vi "Pressure_3_R1.vi"() -> ()   [LabVIEW 2020]
uses:
  Support/Controls/Cmd_Mouse Popup.ctl
  Support/Controls/Clst_Initialize Input.ctl
  Support/Controls/Clst_Result inspec.ctl
  Support/Controls/Cmd_Var Data IO.ctl
  Variables/Global_Cal Info.vi
panel:
  in  "기준온도":string="15" caption="유체기준온도"
  in  "유체":string(combo)="담수"
  in  "Measured_ADJ":string[][](table) caption="Measured (조정후)"
  out "최고수심 (m)":string
  out "Form":string[][](table)
  in  "교정방법":string(combo)="기본교정"
  out "Resolution":string[][](table) caption="Spec"
  in  "지시형태":string(combo)="Check"
  in  "Spec 변경":bool
  in  "Random":bool
  out "Spec":string[][](table)
  out "제목":string
  out "에러 출력":errorcluster
  out "Condition":string[][](table)
  in  "최소눈금 (m)":string(combo)
  out "최대용량 (kPa)":string
  in  "Measured":string[][](table) caption="Measured (조정전)"
  out "Load?":bool
  # "℃"
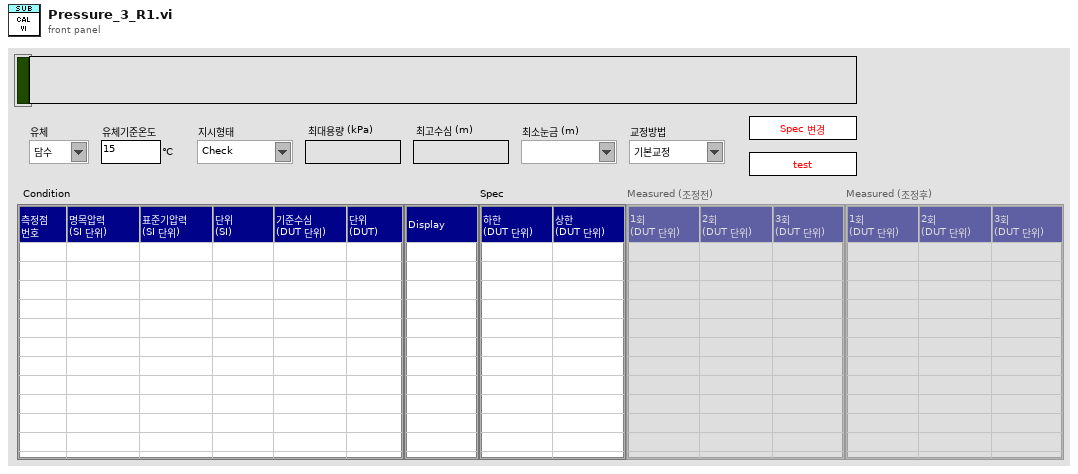
[diagram p1: front panel]
types:
  T1 = typedef "Cmd_Mouse Popup.ctl" = enum16{"활성화", "메뉴선택"}
  T2 = cluster{"Shift":bool, "Ctrl":bool, "Alt":bool, "Cmd":bool, "Opt":bool}
  T3 = enum8{"Enabled", "Disabled", "Disabled and Grayed Out"}
  T4 = cluster{"DisabledEnum":enum8{"Enabled", "Disabled", "Disabled and Grayed Out"}, "Value":string[][], "DisabledEnum":enum8{"Enabled", "Disabled", "Disabled and Grayed Out"}, "Value":string[][], "지시형태":string}
  T5 = typedef "Clst_Initialize Input.ctl" = cluster{"Initialize 1":cluster{"Condition":refnum<vi>[], "Spec":refnum<vi>[], "Measured":refnum<vi>[], "Resolution":refnum<vi>[], "Func_ext":string, "제목":refnum<vi>, "Measured_ADJ":refnum<vi>[]}, "Initialize 2":cluster{"문자열":refnum<vi>[], "콤보박스":refnum<vi>[], "링":refnum<vi>[], "열거형":refnum<vi>[], "테이블":refnum<vi>[], "여러열":refnum<vi>[], "디지털(DBL)":refnum<vi>[], "3D string":refnum<vi>[], "ctrl":refnum<vi>[], "boolean":refnum<vi>[]}}
  T6 = typedef "Clst_Result inspec.ctl" = cluster{"분해능":string, "문자열 1":string, "문자열 2":string, "숫자형 1":i32, "숫자형 2":i32, "숫자형 3":dbl, "문자배열 1D":string[], "문자배열 2D":string[][], "문자배열 3D":string[][][], "문자배열 4D":string[][][][], "불리언 1D":bool[]}
  T7 = typedef "Cmd_Var Data IO.ctl" = enum16{"Condition", "Condition Default", "Condition_Temp", "Resolution", "Resolution Default", "Resolution Old", "Spec", "Spec Default", "Spec Old", "Spec Temp", "Result", "Result2", "Result3", "Result_Temp", "Result_ADJ", "Result_ADJ2", "STD1", "STD2", "STD3", "STD4", "STD5", "STD Temp", "CMC", "CMC Default"}
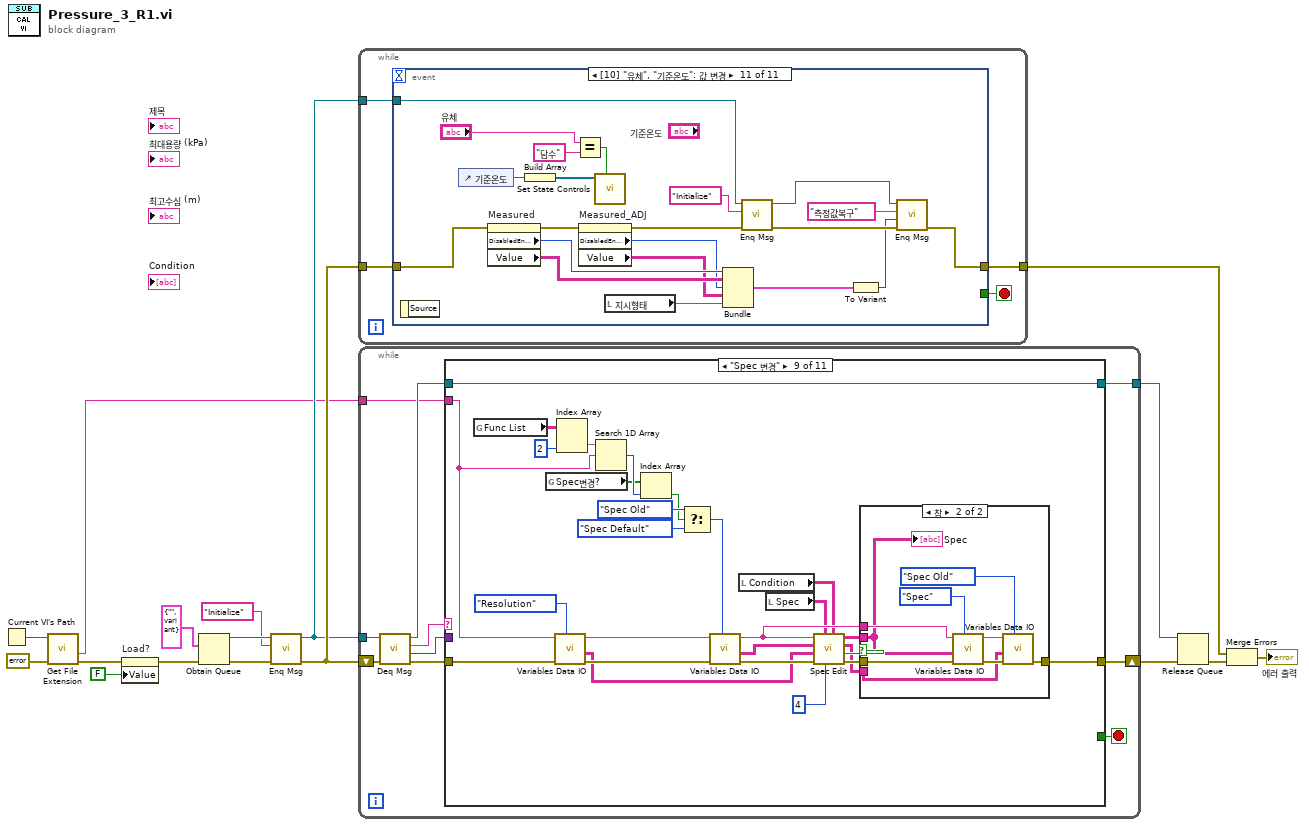
[diagram p0: block diagram]
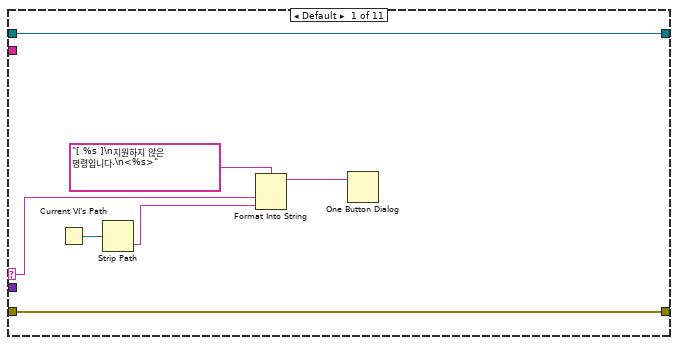
[diagram p2: hidden frame]
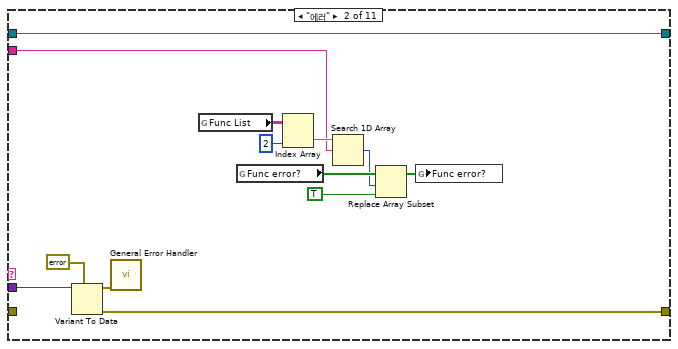
[diagram p3: hidden frame]
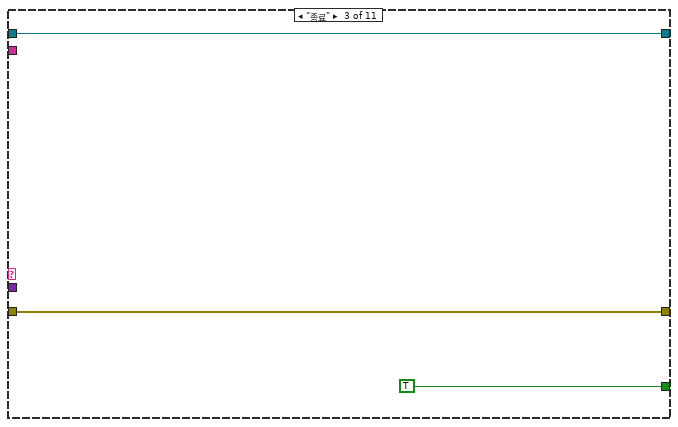
[diagram p4: hidden frame]
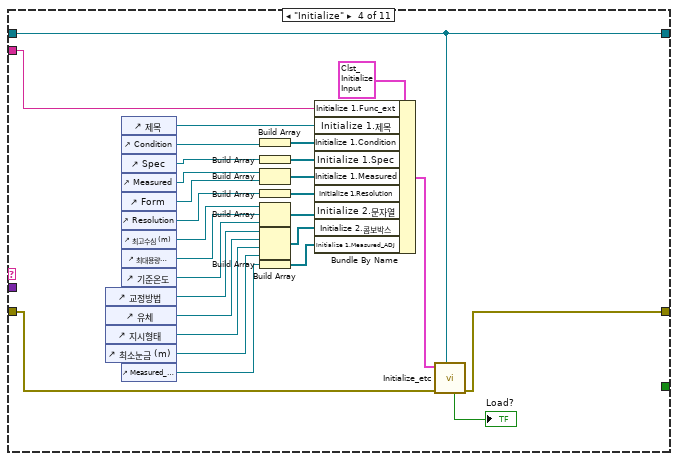
[diagram p5: hidden frame]
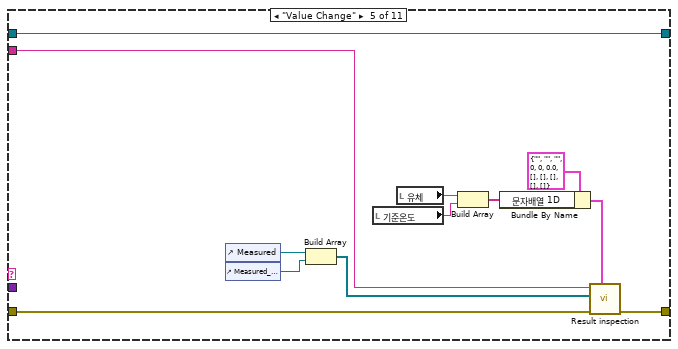
[diagram p6: hidden frame]
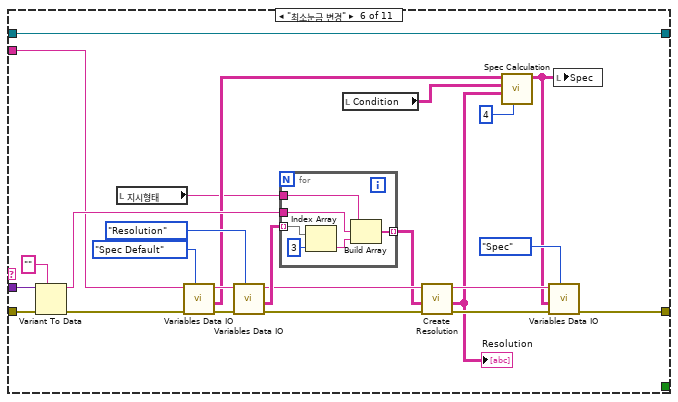
[diagram p7: hidden frame]
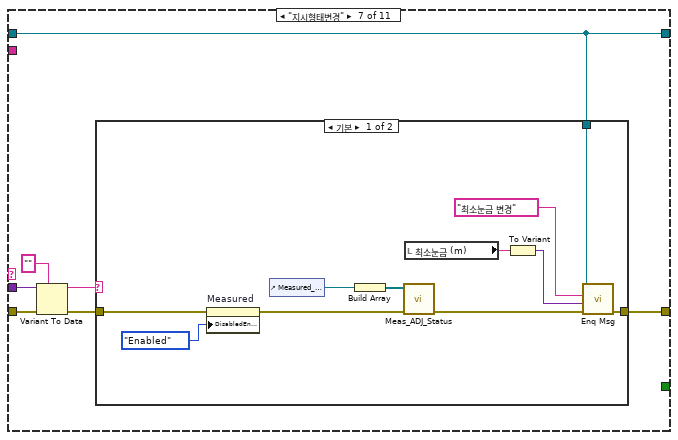
[diagram p8: hidden frame]
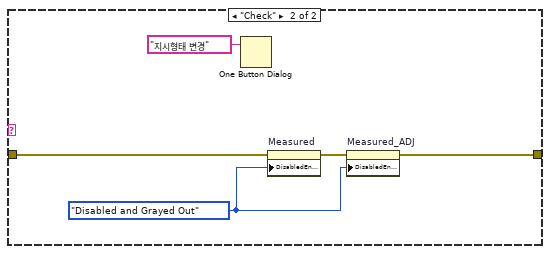
[diagram p9: hidden frame]
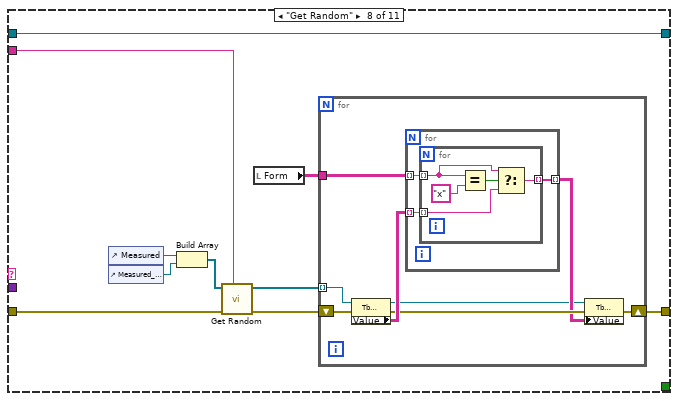
[diagram p10: hidden frame]
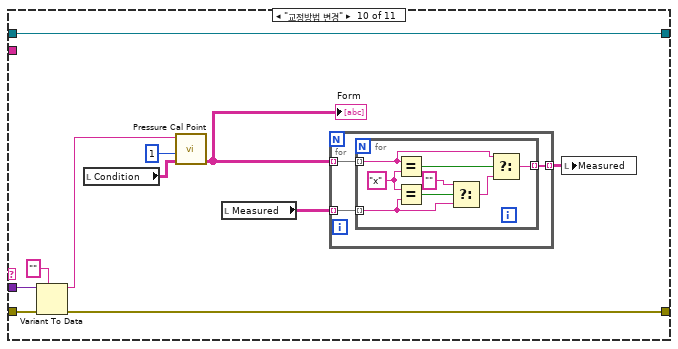
[diagram p12: hidden frame]
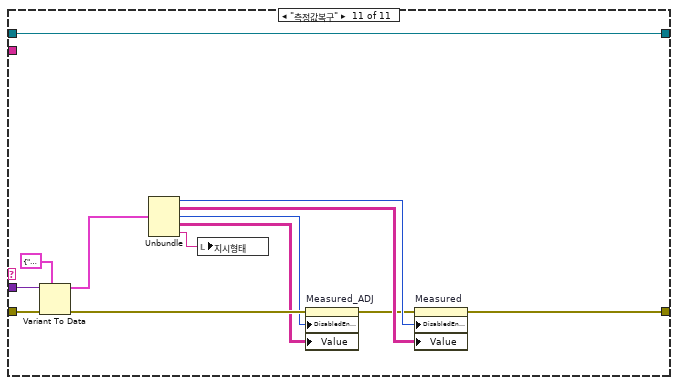
[diagram p13: hidden frame]
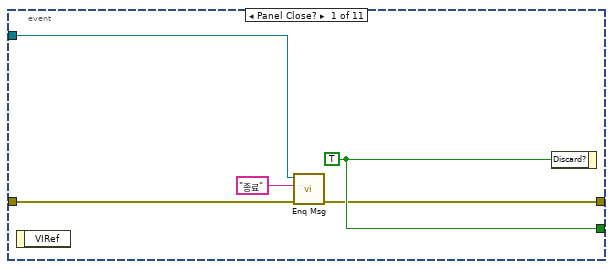
[diagram p14: hidden frame]
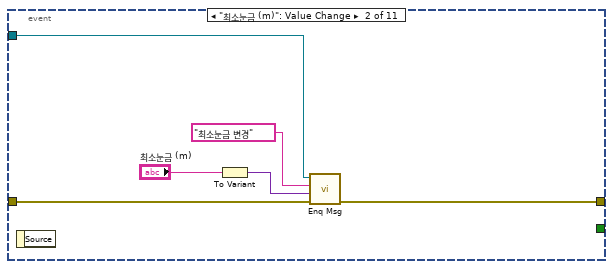
[diagram p15: hidden frame]
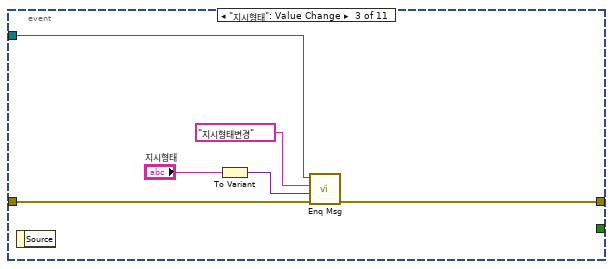
[diagram p16: hidden frame]
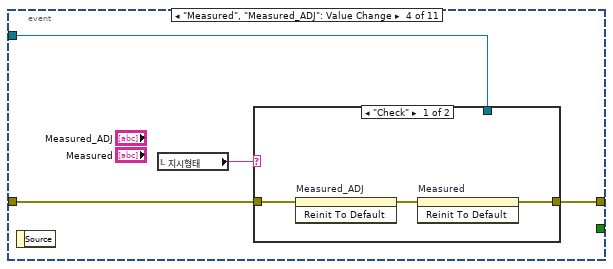
[diagram p17: hidden frame]
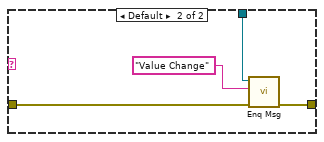
[diagram p18: hidden frame]
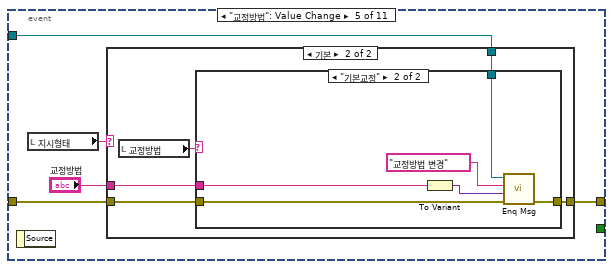
[diagram p19: hidden frame]
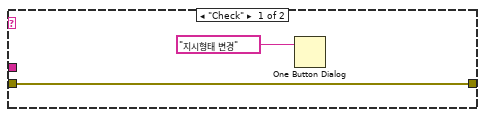
[diagram p20: hidden frame]
diagram:
  n1 = Current VI's Path() -> (path=w5:path)
  n2 = call <vilib>:"Get File Extension.vi"("error in (no error)"=errorcluster {"status"=FALSE, "code"=0, "source"=""} ("에러 상수"), "file"=w5) -> ("error out"=w2:errorcluster, "filename without extension"=w4:string)  [unwired: 5 in, 3 out]
  n3 = property on="Load?" class="Bool (엄격한)"(error in=w2, "Value"=FALSE ("Load?")) -> (error out=w1:errorcluster)  [unwired: 1 in, 1 out]
  n4 = Obtain Queue(element data type=cluster{"메세지":string, "값":variant} {"메세지"="", "값"=variant} ("Message Cluster"), error in (no error)=w1) -> (queue out=w14:refnum<queue>, error out=w16:errorcluster)  [unwired: 3 in, 1 out]
  n5 = call "Enq Msg.vi"("에러 입력(에러 없음)"=w16, "메세지"="Initialize", "큐 입력"=w14) -> ("에러 출력"=w15:errorcluster, "큐 출력"=w12:refnum<queue>)  [unwired: 7 in]
  n6 = while {
    tunnel: w15 -> [w19]
    tunnel: w12 -> [w20]
    tunnel: [w18] -> w9
    stop <- w21 stop-if-true
    n7 = event shown="[10] \"유체\", \"기준온도\": 값 변경" {
      selector: _ -> [_ _ _ _ _ _ _ _ _ _ _]
      dyn-events: _ -> [_ _ _ _ _ _ _ _ _ _ _]
      timeout: _ -> [_ _ _ _ _ _ _ _ _ _ _]
      tunnel: [w26 _ _ _ _ _ _ _ _ _ _] -> w21
      tunnel: w20 -> [w24 w31 w37 w41 w50 _ w90 _ w103 w109 w127]
      tunnel: w19 -> [w25 w32 w38 w42 w53 w86 w94 w101 w104 w111 w121]
      tunnel: [w22 w30 w36 w40 w54 w85 w89 w100 w102 w110 w124] -> w18
      event Panel Close? {
        w26 = TRUE ("버림?")
        n8 = event-data() -> ()  [unwired: 1 in, 1 out]
        n9 = call "Enq Msg.vi"("에러 입력(에러 없음)"=w25, "메세지"="종료", "큐 입력"=w24) -> ("에러 출력"=w22:errorcluster)  [unwired: 7 in, 1 out]
        n10 = event-data("Discard?"=w26) -> ()  [unwired: 1 in, 1 out]
      }
      event "최소눈금 (m)": Value Change {
        n11 = event-data() -> ()  [unwired: 1 in, 1 out]
        n12 = To Variant(anything="최소눈금 (m)") -> (Variant=w27:variant)
        n13 = call "Enq Msg.vi"("에러 입력(에러 없음)"=w32, "값"=w27, "메세지"="최소눈금 변경", "큐 입력"=w31) -> ("에러 출력"=w30:errorcluster)  [unwired: 6 in, 1 out]
      }
      event "지시형태": Value Change {
        n14 = event-data() -> ()  [unwired: 1 in, 1 out]
        n15 = To Variant(anything="지시형태") -> (Variant=w34:variant)
        n16 = call "Enq Msg.vi"("에러 입력(에러 없음)"=w38, "값"=w34, "메세지"="지시형태변경", "큐 입력"=w37) -> ("에러 출력"=w36:errorcluster)  [unwired: 6 in, 1 out]
      }
      event "Measured", "Measured_ADJ": Value Change {
        n17 = event-data() -> ()  [unwired: 1 in, 1 out]
        n18 = local read "지시형태"() -> (w39:string)
        n19 = case shown="\"Check\"" w39 {
          tunnel: w42 -> [w45 w49]
          tunnel: w41 -> [_ w48]
          tunnel: [w43 w47] -> w40
          frame "Check" {
            n20 = invoke on="Measured_ADJ" class="Tbl (엄격한)" method="Reinit To Default"(error in=w45) -> (error out=w44:errorcluster)  [unwired: 2 in, 2 out]
            n21 = invoke on="Measured" class="Tbl (엄격한)" method="Reinit To Default"(error in=w44) -> (error out=w43:errorcluster)  [unwired: 2 in, 2 out]
          }
          frame Default {
            n22 = call "Enq Msg.vi"("에러 입력(에러 없음)"=w49, "메세지"="Value Change", "큐 입력"=w48) -> ("에러 출력"=w47:errorcluster)  [unwired: 7 in, 1 out]
          }
        }
      }
      event "교정방법": Value Change {
        n23 = event-data() -> ()  [unwired: 1 in, 1 out]
        n24 = local read "지시형태"() -> (w51:string)
        n25 = case shown="기본" w51 {
          tunnel: w53 -> [w56 w61]
          tunnel: w50 -> [_ w60]
          tunnel: [w56 w59] -> w54
          tunnel: "교정방법" -> [_ w58]
          frame "Check" {
            n26 = One Button Dialog(message="지시형태 변경" ("메시지")) -> ()  [unwired: 1 in, 1 out]
          }
          frame Default {
            n27 = local read "교정방법"() -> (w57:string)
            n28 = case shown="\"기본교정\"" w57 {
              tunnel: w61 -> [w68 w83]
              tunnel: w60 -> [w67 w82]
              tunnel: [w66 w81] -> w59
              tunnel: w58 -> [w65 w80]
              frame Default {
                n29 = local read "Condition"() -> (w62:string[][])
                n30 = Array Size(array=w62) -> (size(s)=w64:i32[])
                n31 = Index Array(array=w64) -> (element=w63:i32)  [unwired: 1 in]
                n32 = case shown="기본" w63 {
                  tunnel: w68 -> [w71 w77]
                  tunnel: w67 -> [_ w76]
                  tunnel: [w71 w74] -> w66
                  tunnel: w65 -> [_ w72]
                  frame 0..21 {
                    n33 = local write "교정방법"("기본교정" ("교정방법")) -> ()
                    n34 = One Button Dialog(message="표준, 종합 교정은 11 측정점 이상 가능" ("메시지")) -> ()  [unwired: 1 in, 1 out]
                  }
                  frame Default {
                    n35 = To Variant(anything=w72) -> (Variant=w73:variant)
                    n36 = call "Enq Msg.vi"("에러 입력(에러 없음)"=w77, "값"=w73, "메세지"="교정방법 변경", "큐 입력"=w76) -> ("에러 출력"=w74:errorcluster)  [unwired: 6 in, 1 out]
                  }
                }
              }
              frame "기본교정" {
                n37 = To Variant(anything=w80) -> (Variant=w78:variant)
                n38 = call "Enq Msg.vi"("에러 입력(에러 없음)"=w83, "값"=w78, "메세지"="교정방법 변경", "큐 입력"=w82) -> ("에러 출력"=w81:errorcluster)  [unwired: 6 in, 1 out]
              }
            }
          }
        }
      }
      event "Condition", "Spec", "Measured", "Measured_ADJ": Shortcut Menu Activation? {
        n39 = event-data() -> ("MenuRef"=w84:refnum<k9>)  [unwired: 1 in]
        n40 = call "Mouse PopUp Control.vi"("type"=Cmd_Mouse_Popup."활성화", "error in"=w86, "메뉴 참조"=w84) -> ("error out"=w85:errorcluster)  [unwired: 8 in]
        n41 = event-data() -> ()  [unwired: 2 in, 1 out]
      }
      event "Condition", "Spec", "Measured", "Measured_ADJ": Shortcut Menu Selection (User) {
        n42 = event-data() -> ("CtlRef"=w92:refnum<vi>, "ItemTag"=w93:string)  [unwired: 1 in]
        n43 = call "Mouse PopUp Control.vi"("type"=Cmd_Mouse_Popup."메뉴선택", "error in"=w94, "아이템 태그"=w93, "Tbl 참조 번호"=w92) -> ("error out"=w91:errorcluster)  [unwired: 7 in]
        n44 = call "Enq Msg.vi"("에러 입력(에러 없음)"=w91, "메세지"="Value Change", "큐 입력"=w90) -> ("에러 출력"=w89:errorcluster)  [unwired: 7 in, 1 out]
      }
      event "Measured", "Condition", "Measured_ADJ": Key Down; "Measured", "Condition", "Measured_ADJ": Key Repeat {
        n45 = event-data() -> ("PlatMods"=w96:T2, "ScanCode"=w99:i16, "Mods.Num Pad"=w98:bool, "CtlRef"=w97:refnum<vi>)  [unwired: 1 in]
        n46 = call "Cursor Control.vi"("플랫폼 조합키"=w96, "참조"=w97, "Num Pad"=w98, "ScanCode"=w99, "error in"=w101) -> ("error out"=w100:errorcluster)  [unwired: 5 in, 1 out]
      }
      event "Random": Value Change {
        n47 = event-data() -> ()  [unwired: 1 in, 1 out]
        n48 = call "Enq Msg.vi"("에러 입력(에러 없음)"=w104, "메세지"="Get Random", "큐 입력"=w103) -> ("에러 출력"=w106:errorcluster, "큐 출력"=w107:refnum<queue>)  [unwired: 7 in]
        n49 = call "Enq Msg.vi"("에러 입력(에러 없음)"=w106, "메세지"="Value Change", "큐 입력"=w107) -> ("에러 출력"=w102:errorcluster)  [unwired: 7 in, 1 out]
      }
      event "Spec 변경": Value Change {
        n50 = event-data() -> ()  [unwired: 1 in, 1 out]
        n51 = call "Enq Msg.vi"("에러 입력(에러 없음)"=w111, "메세지"="Spec 변경", "큐 입력"=w109) -> ("에러 출력"=w110:errorcluster)  [unwired: 7 in, 1 out]
      }
      event "유체", "기준온도": Value Change {
        n52 = event-data() -> ()  [unwired: 1 in, 1 out]
        n53 = control-ref of="기준온도"() -> (w133:refnum<vi>)
        n54 = property on="Measured" class="Tbl (엄격한)"(error in=w121) -> (error out=w120:errorcluster, "DisabledEnum"=w118:T3, "Value"=w117:string[][])  [unwired: 1 in, 1 out]
        n55 = Build Array(w133) -> (w132:refnum<vi>[])
        n56 = Equal?(x="유체", y="담수") -> (x = y?=w129:bool)
        n57 = property on="Measured_ADJ" class="Tbl (엄격한)"(error in=w120) -> (error out=w119:errorcluster, "DisabledEnum"=w116:T3, "Value"=w115:string[][])  [unwired: 1 in, 1 out]
        n58 = call "Set State Controls.vi"("활성화 (F)"=w129, "컨트롤 참조 배열 in"=w132) -> ()  [unwired: 8 in, 2 out]
        n59 = local read "지시형태"() -> (w114:string)
        n60 = Bundle("DisabledEnum"=w118, "Value"=w117, "DisabledEnum"=w116, "Value"=w115, "지시형태"=w114) -> (w113:T4)  [unwired: 1 in]
        n61 = call "Enq Msg.vi"("에러 입력(에러 없음)"=w119, "메세지"="Initialize", "큐 입력"=w127) -> ("에러 출력"=w125:errorcluster, "큐 출력"=w123:refnum<queue>)  [unwired: 7 in]
        n62 = To Variant(anything=w113) -> (Variant=w122:variant)
        n63 = call "Enq Msg.vi"("에러 입력(에러 없음)"=w125, "값"=w122, "메세지"="측정값복구", "큐 입력"=w123) -> ("에러 출력"=w124:errorcluster)  [unwired: 6 in, 1 out]
      }
    }
  }
  n64 = while {
    shift-right: [w143] -> w11
    shift-left: w15 -> [w142]
    tunnel: w12 -> [w140]
    tunnel: [w135] -> w10
    tunnel: w4 -> [w134]
    stop <- w136 stop-if-true
    n65 = call "Deq Msg.vi"("에러 입력(에러 없음)"=w142, "큐 입력"=w140) -> ("에러 출력"=w141:errorcluster, "값"=w137:variant, "메세지"=w139:string, "큐 출력"=w138:refnum<queue>)  [unwired: 6 in]
    n66 = case shown="\"Spec 변경\"" w139 {
      selector: w139 -> [w146 _ _ _ _ _ _ _ _ _ _]
      tunnel: w141 -> [w150 _ w166 w181 w203 w229 w243 w268 w307 w331 w357]
      tunnel: [w150 w160 w166 w177 w205 w211 w239 w263 w311 w330 w346] -> w143
      tunnel: w138 -> [w149 w159 w164 w182 w206 w231 w238 w270 w313 w334 w358]
      tunnel: w137 -> [_ w161 _ _ _ w228 w242 _ _ w332 w356]
      tunnel: [_ _ TRUE ("버림?") _ _ _ _ _ _ _ _] -> w136
      tunnel: [w149 w159 w164 w182 w206 w231 w238 w270 w313 w334 w358] -> w135
      tunnel: w134 -> [_ w151 _ w176 w204 w221 _ w266 w288 _ _]
      frame Default {
        n67 = Current VI's Path() -> (path=w145:path)
        n68 = Strip Path(path=w145) -> (name=w144:string)  [unwired: 1 out]
        n69 = Format Into String(format string="[ %s ]\n지원하지 않은 명령입니다.\n<%s>" ("메시지"), w146, w144) -> (resulting string=w147:string)  [unwired: 2 in, 1 out]
        n70 = One Button Dialog(message=w147) -> ()  [unwired: 1 in, 1 out]
      }
      frame "에러" {
        n71 = Variant To Data(type=errorcluster {"status"=FALSE, "code"=0, "source"=""} ("에러 출력"), Variant=w161) -> (data=w163:errorcluster, error out=w160:errorcluster)  [unwired: 1 in]
        n72 = call <vilib>:"General Error Handler.vi"("error in (no error)"=w163) -> ()  [unwired: 10 in, 5 out]
        n73 = global read "Global_Cal Info.vi" "Func List"() -> (w157:string[][])
        n74 = global read "Global_Cal Info.vi" "Func error?"() -> (w154:bool[])
        n75 = Index Array(array=w157, index (col)=2 ("비활성화된 인덱스 (열)")) -> (element=w156:string[])  [unwired: 1 in]
        n76 = Search 1D Array(1D array=w156, element=w151) -> (index of element=w153:i32)  [unwired: 1 in]
        n77 = Replace Array Subset(array=w154, new element=TRUE ("새 원소/부분배열"), index=w153) -> (w152:bool[])
        n78 = global write "Global_Cal Info.vi" "Func error?"(w152) -> ()
      }
      frame "종료" {
      }
      frame "Initialize" {
        n79 = control-ref of="교정방법"() -> (w170:refnum<vi>)
        n80 = control-ref of="유체"() -> (w169:refnum<vi>)
        n81 = control-ref of="지시형태"() -> (w168:refnum<vi>)
        n82 = control-ref of="최소눈금 (m)"() -> (w167:refnum<vi>)
        n83 = control-ref of="제목"() -> (w186:refnum<vi>)
        n84 = control-ref of="Condition"() -> (w192:refnum<vi>)
        n85 = control-ref of="Spec"() -> (w184:refnum<vi>)
        n86 = control-ref of="Measured"() -> (w189:refnum<vi>)
        n87 = control-ref of="Form"() -> (w178:refnum<vi>)
        n88 = control-ref of="Resolution"() -> (w180:refnum<vi>)
        n89 = control-ref of="최고수심 (m)"() -> (w185:refnum<vi>)
        n90 = control-ref of="최대용량 (kPa)"() -> (w175:refnum<vi>)
        n91 = control-ref of="기준온도"() -> (w171:refnum<vi>)
        n92 = control-ref of="Measured_ADJ"() -> (w173:refnum<vi>)
        n93 = Build Array(w192) -> (w191:refnum<vi>[])
        n94 = Build Array(w184) -> (w183:refnum<vi>[])
        n95 = Build Array(w189, w178) -> (w190:refnum<vi>[])
        n96 = Build Array(w180) -> (w179:refnum<vi>[])
        n97 = Build Array(w185, w175, w171) -> (w188:refnum<vi>[])
        n98 = Build Array(w170, w169, w168, w167) -> (w187:refnum<vi>[])
        n99 = Build Array(w173) -> (w174:refnum<vi>[])
        n100 = Bundle By Name(cluster=T5 {"Initialize 1"={"Condition"=[], "Spec"=[], "Measured"=[], "Resolution"=[], "Func_ext"="", "제목"=refnum, "Measured_ADJ"=[]}, "Initialize 2"={"문자열"=[], "콤보박스"=[], "링"=[], "열거형"=[], "테이블"=[], "여러열"=[], "디지털(DBL)"=[], "3D string"=[], "ctrl"=[], "boolean"=[]}} ("입력 클러스터"), "Initialize 1.Func_ext"=w176, "Initialize 1.제목"=w186, "Initialize 1.Condition"=w191, "Initialize 1.Spec"=w183, "Initialize 1.Measured"=w190, "Initialize 1.Resolution"=w179, "Initialize 2.문자열"=w188, "Initialize 2.콤보박스"=w187, "Initialize 1.Measured_ADJ"=w174) -> (w193:T5)
        n101 = call "Initialize_etc.vi"("큐 입력"=w182, "error in"=w181, "입력 클러스터"=w193) -> ("error out"=w177:errorcluster, "Load?"=→"Load?":bool)  [unwired: 6 in, 1 out]
      }
      frame "Value Change" {
        n102 = control-ref of="Measured"() -> (w202:refnum<vi>)
        n103 = control-ref of="Measured_ADJ"() -> (w200:refnum<vi>)
        n104 = Build Array(w202, w200) -> (w201:refnum<vi>[])
        n105 = local read "기준온도"() -> (w195:string)
        n106 = local read "유체"() -> (w199:string)
        n107 = Build Array(w199, w195) -> (w197:string[])
        n108 = Bundle By Name(cluster=T6 {"분해능"="", "문자열 1"="", "문자열 2"="", "숫자형 1"=0, "숫자형 2"=0, "숫자형 3"=0.0, "문자배열 1D"=[], "문자배열 2D"=[], "문자배열 3D"=[], "문자배열 4D"=[], "불리언 1D"=[]} ("입력 클러스터"), "문자배열 1D"=w197) -> (w196:T6)
        n109 = call "Result inspection.vi"("입력 클러스터"=w196, "error in"=w203, "Ref. Data (Inspection)"=w201, "Func ext"=w204) -> ("error out"=w205:errorcluster)  [unwired: 4 in, 3 out]
      }
      frame "최소눈금 변경" {
        n110 = Variant To Data(error in=w229, type="", Variant=w228) -> (data=w226:string, error out=w222:errorcluster)
        n111 = local read "지시형태"() -> (w207:string)
        n112 = call "Variables Data IO.vi"("Select"=Cmd_Var_Data_IO."Spec Default", "error in"=w222, "Func_ext"=w221) -> ("error out"=w219:errorcluster, "Data Out"=w217:string[][], "Func_ext Out"=w220:string)  [unwired: 6 in]
        n113 = call "Variables Data IO.vi"("Select"=Cmd_Var_Data_IO."Resolution", "error in"=w219, "Func_ext"=w220) -> ("error out"=w224:errorcluster, "Data Out"=w230:string[][], "Func_ext Out"=w223:string)  [unwired: 6 in]
        n114 = for {
          tunnel: w230 -> [w237] mode=indexing
          tunnel: w226 -> [w236]
          tunnel: [w234] -> w209 mode=indexing
          tunnel: w207 -> [w233]
          n115 = Index Array(array=w237, index=3 ("인덱스")) -> (element=w235:string)
          n116 = Build Array(w233, w236, w235) -> (w234:string[])
        }
        n117 = local read "Condition"() -> (w216:string[][])
        n118 = call "Create Resolution.vi"("에러 입력(에러 없음)"=w224, "Resolution"=w209, "Func_ext"=w223) -> ("에러 출력"=w212:errorcluster, "Resolution Out"=w208:string[][], "Func_ext 출력"=w213:string)  [unwired: 6 in]
        "Resolution" <- w208
        n119 = call "Spec Calculation.vi"("기준값 열번호"=4 ("열번호(기준값)"), "Resolution"=w208, "Condition in"=w216, "Spec Default"=w217) -> ("Spec out"=w210:string[][])  [unwired: 6 in, 1 out]
        n120 = call "Variables Data IO.vi"("Select"=Cmd_Var_Data_IO."Spec", "error in"=w212, "Data In"=w210, "Func_ext"=w213) -> ("error out"=w211:errorcluster)  [unwired: 5 in, 2 out]
        n121 = local write "Spec"(w210) -> ()
      }
      frame "지시형태변경" {
        n122 = Variant To Data(error in=w243, type="", Variant=w242) -> (data=w241:string, error out=w240:errorcluster)
        n123 = case shown="기본" w241 {
          tunnel: w240 -> [w255 w260]
          tunnel: [w247 w258] -> w239
          tunnel: w238 -> [w246 _]
          frame Default {
            n124 = property on="Measured" class="Tbl (엄격한)"(error in=w255, "DisabledEnum"=T3."Enabled" ("비활성화")) -> (error out=w252:errorcluster)  [unwired: 1 in, 1 out]
            n125 = control-ref of="Measured_ADJ"() -> (w251:refnum<vi>)
            n126 = Build Array(w251) -> (w253:refnum<vi>[])
            n127 = call "Meas_ADJ_Status.vi"("에러 입력(에러 없음)"=w252, "Measured_ADJ in"=w253) -> ("에러 출력"=w248:errorcluster)  [unwired: 8 in, 1 out]
            n128 = local read "최소눈금 (m)"() -> (w245:string)
            n129 = To Variant(anything=w245) -> (Variant=w250:variant)
            n130 = call "Enq Msg.vi"("에러 입력(에러 없음)"=w248, "값"=w250, "메세지"="최소눈금 변경", "큐 입력"=w246) -> ("에러 출력"=w247:errorcluster)  [unwired: 6 in, 1 out]
          }
          frame "Check" {
            w257 = T3."Disabled and Grayed Out" ("비활성화")
            n131 = One Button Dialog(message="지시형태 변경" ("메시지")) -> ()  [unwired: 1 in, 1 out]
            n132 = property on="Measured" class="Tbl (엄격한)"(error in=w260, "DisabledEnum"=w257) -> (error out=w259:errorcluster)  [unwired: 1 in, 1 out]
            n133 = property on="Measured_ADJ" class="Tbl (엄격한)"(error in=w259, "DisabledEnum"=w257) -> (error out=w258:errorcluster)  [unwired: 1 in, 1 out]
          }
        }
      }
      frame "Get Random" {
        n134 = control-ref of="Measured"() -> (w267:refnum<vi>)
        n135 = control-ref of="Measured_ADJ"() -> (w262:refnum<vi>)
        n136 = Build Array(w267, w262) -> (w269:refnum<vi>[])
        n137 = call "Get Random.vi"("Func_Ext"=w266, "에러 입력"=w268, "Meas"=w269) -> ("에러 출력"=w265:errorcluster, "Meas out"=w261:refnum<vi>[])  [unwired: 7 in]
        n138 = local read "Form"() -> (w264:string[][])
        n139 = for {
          tunnel: w264 -> [w277]
          shift-right: [w274] -> w263
          shift-left: w265 -> [w278]
          tunnel: w261 -> [w271] mode=indexing
          n140 = property on="프로퍼티 노드" class="Tbl (엄격한)"(reference=w271, error in=w278) -> (reference out=w272:refnum<vi>, error out=w275:errorcluster, "Value"=w276:string[][])
          n141 = for {
            tunnel: w277 -> [w281] mode=indexing
            tunnel: w276 -> [w280] mode=indexing
            tunnel: [w279] -> w273 mode=indexing
            n142 = for {
              tunnel: w281 -> [w284] mode=indexing
              tunnel: w280 -> [w283] mode=indexing
              tunnel: [w282] -> w279 mode=indexing
              n143 = Equal?(x=w284, y="ⅹ") -> (x = y?=w285:bool)
              n144 = Select(t=w284, s=w285, f=w283) -> (s? t:f=w282:string)
            }
          }
          n145 = property on="프로퍼티 노드" class="Tbl (엄격한)"(reference=w272, error in=w275, "Value"=w273) -> (error out=w274:errorcluster)  [unwired: 1 out]
        }
      }
      frame "Spec 변경" {
        n146 = global read "Global_Cal Info.vi" "Func List"() -> (w293:string[][])
        n147 = global read "Global_Cal Info.vi" "Spec변경?"() -> (w289:bool[])
        n148 = call "Variables Data IO.vi"("Select"=Cmd_Var_Data_IO."Resolution", "error in"=w307, "Func_ext"=w288) -> ("error out"=w306:errorcluster, "Data Out"=w300:string[][], "Func_ext Out"=w305:string)  [unwired: 6 in]
        n149 = Index Array(array=w293, index (col)=2 ("비활성화된 인덱스 (열)")) -> (element=w291:string[])  [unwired: 1 in]
        n150 = Search 1D Array(1D array=w291, element=w288) -> (index of element=w290:i32)  [unwired: 1 in]
        n151 = Index Array(array=w289, index=w290) -> (element=w294:bool)
        n152 = Select(t=Cmd_Var_Data_IO."Spec Old" ("Select"), s=w294, f=Cmd_Var_Data_IO."Spec Default" ("Select")) -> (s? t:f=w287:T7)
        n153 = call "Variables Data IO.vi"("Select"=w287, "error in"=w306, "Func_ext"=w305) -> ("error out"=w308:errorcluster, "Data Out"=w299:string[][], "Func_ext Out"=w301:string)  [unwired: 6 in]
        n154 = local read "Condition"() -> (w297:string[][])
        n155 = local read "Spec"() -> (w298:string[][])
        n156 = call "Spec Edit.vi"("Condition"=w297, "열번호(기준값)"=4 ("기준열(0)"), "Spec Value"=w298, "에러 입력(에러 없음)"=w308, "Resolution"=w300, "Spec Default"=w299, "Func_ext"=w301) -> ("에러 출력"=w312:errorcluster, "변경?"=w309:bool, "Spec Default out"=w303:string[][], "Spec 출력"=w310:string[][])  [unwired: 1 in]
        n157 = case shown="참" w309 {
          tunnel: w312 -> [w314 w322]
          tunnel: [w314 w318] -> w311
          tunnel: w310 -> [_ w320]
          tunnel: w301 -> [_ w321]
          tunnel: w303 -> [_ w316]
          frame False {
          }
          frame True {
            n158 = call "Variables Data IO.vi"("Select"=Cmd_Var_Data_IO."Spec", "error in"=w322, "Data In"=w320, "Func_ext"=w321) -> ("error out"=w319:errorcluster, "Func_ext Out"=w317:string)  [unwired: 5 in, 1 out]
            n159 = call "Variables Data IO.vi"("Select"=Cmd_Var_Data_IO."Spec Old", "error in"=w319, "Data In"=w316, "Func_ext"=w317) -> ("error out"=w318:errorcluster)  [unwired: 5 in, 2 out]
            "Spec" <- w320
          }
        }
      }
      frame "교정방법 변경" {
        n160 = Variant To Data(error in=w331, type="", Variant=w332) -> (data=w327:string, error out=w330:errorcluster)
        n161 = local read "Condition"() -> (w326:string[][])
        n162 = call "Pressure Cal Point.vi"("Condition"=w326, "인덱스 (열)"=1, "교정방법"=w327) -> ("배열"=w324:string[][])  [unwired: 5 in, 3 out]
        "Form" <- w324
        n163 = local read "Measured"() -> (w329:string[][])
        n164 = for {
          tunnel: w324 -> [w337] mode=indexing
          tunnel: w329 -> [w336] mode=indexing
          tunnel: [w335] -> w328 mode=indexing
          n165 = for {
            tunnel: w337 -> [w344] mode=indexing
            tunnel: w336 -> [w340] mode=indexing
            tunnel: [w338] -> w335 mode=indexing
            w343 = "ⅹ"
            n166 = Equal?(x=w344, y=w343) -> (x = y?=w345:bool)
            n167 = Equal?(x=w343, y=w340) -> (x = y?=w342:bool)
            n168 = Select(t="", s=w342, f=w340) -> (s? t:f=w339:string)
            n169 = Select(t=w344, s=w345, f=w339) -> (s? t:f=w338:string)
          }
        }
        n170 = local write "Measured"(w328) -> ()
      }
      frame "측정값복구" {
        n171 = Variant To Data(error in=w357, type=T4 {"DisabledEnum"=enum."Enabled", "Value"=[], "DisabledEnum"=enum."Enabled", "Value"=[], "지시형태"=""} ("출력 클러스터"), Variant=w356) -> (data=w354:T4, error out=w350:errorcluster)
        n172 = Unbundle(w354) -> ("DisabledEnum"=w353:T3, "Value"=w352:string[][], "DisabledEnum"=w349:T3, "Value"=w348:string[][], "지시형태"=w347:string)
        n173 = local write "지시형태"(w347) -> ()
        n174 = property on="Measured_ADJ" class="Tbl (엄격한)"(error in=w350, "DisabledEnum"=w349, "Value"=w348) -> (error out=w351:errorcluster)  [unwired: 1 in, 1 out]
        n175 = property on="Measured" class="Tbl (엄격한)"(error in=w351, "DisabledEnum"=w353, "Value"=w352) -> (error out=w346:errorcluster)  [unwired: 1 in, 1 out]
      }
    }
  }
  n176 = Release Queue(queue=w10, error in (no error)=w11) -> (error out=w8:errorcluster)  [unwired: 1 in, 2 out]
  n177 = Merge Errors(w9, w8) -> (→"에러 출력":errorcluster)
